vi "Open Front Panel.vi"(8 "error in (no error)":errorcluster, 11 "reference":refnum<vi>) -> (0 "error out":errorcluster, 3 "reference out":refnum<vi>)   [LabVIEW 2015]
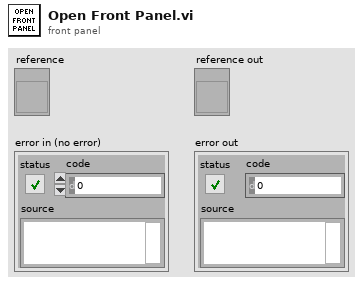
[diagram p1: front panel]
types:
  T1 = enum32{"Invalid", "Standard", "Closed", "Hidden", "Minimized", "Maximized"}
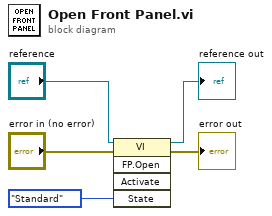
[diagram p0: block diagram]
diagram:
  n1 = invoke class="VI" method="FP.Open"(reference="reference", error in="error in (no error)", "State"=T1."Standard") -> (reference out=→"reference out":refnum<vi>, error out=→"error out":errorcluster)  [unwired: 2 in, 3 out]
